vi "Store Numeric (SubVI).vi"(7 "Commands":T1, 8 "error in":errorcluster, 11 "Primary Numeric":dbl) -> (0 "error out":errorcluster, 2 "No. Stored Elements":i32, 3 "Stored Values":dbl[](array[numeric]))   [LabVIEW 2012]
doc: "FGV to store the numeric values which are used in computation."
uses:
  Controls/Storage Commands.ctl
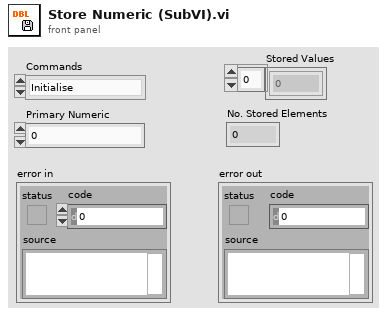
[diagram p1: front panel]
types:
  T1 = typedef "Storage Commands.ctl" = enum16{"Initialise", "Build", "GET", "Reset"}
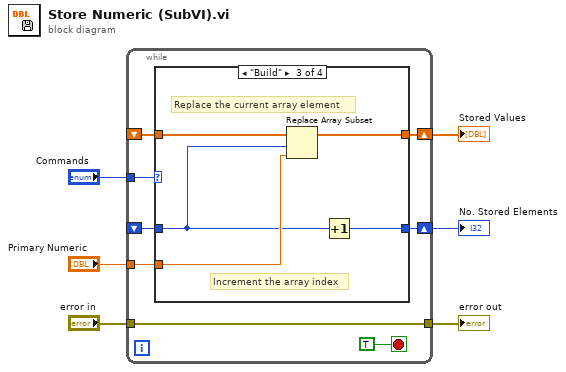
[diagram p0: block diagram]
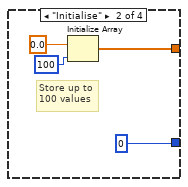
[diagram p3: hidden frame]
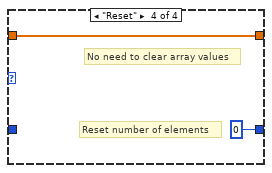
[diagram p4: hidden frame]
diagram:
  n1 = while {
    tunnel: "error in" -> [w14]
    tunnel: [w14] -> w6
    shift-right: [w11] -> w3
    shift-left: _ -> [w10]
    tunnel: "Commands" -> [w12]
    tunnel: "Primary Numeric" -> [w9]
    shift-right: [w8] -> w1
    shift-left: _ -> [w7]
    stop <- TRUE stop-if-true
    n2 = case shown="\"Build\"" w12 {
      tunnel: [w16 w20 w24 w26] -> w11
      tunnel: w10 -> [w16 _ w25 w26]
      tunnel: w9 -> [_ _ w23 _]
      tunnel: [w15 0 ("dimension size") w22 0 ("dimension size")] -> w8
      tunnel: w7 -> [w15 _ w21 _]
      frame "GET" {
        # "Returns the Stored Values array and\nthe number of stored elements"
      }
      frame "Initialise" {
        # "Store up to\n100 values"
        n3 = Initialize Array(0.0, 100 ("dimension size")) -> (w20:dbl[])
      }
      frame "Build" {
        # "Increment the array index"
        # "Replace the current array element"
        n4 = Replace Array Subset(array=w25, new element=w23, index=w21) -> (w24:dbl[])
        n5 = Increment(x=w21) -> (x+1=w22:i32)
      }
      frame "Reset" {
        # "No need to clear array values"
        # "Reset number of elements"
      }
    }
  }
  "error out" <- w6
  "Stored Values" <- w3
  "No. Stored Elements" <- w1
